vi "Stop Server.vi"(8 "error in":errorcluster, 9 "timeout ms (1000)":i32=1000, 10 "abort (F)":bool, 11 "port (0)":u16) -> (0 "error out":errorcluster)   [LabVIEW 2010, in "NI_CCC.lvlib"]
doc: "Stops the CCC server process.\n\nIf the value of <b>port</b> is 0, all instances of the CCC server process will be stopped. Otherwise, only the CCC server process instance corresponding to the port number will be stopped."
uses:
  NI_CCC.lvlib
  FG Server Instances Action.ctl
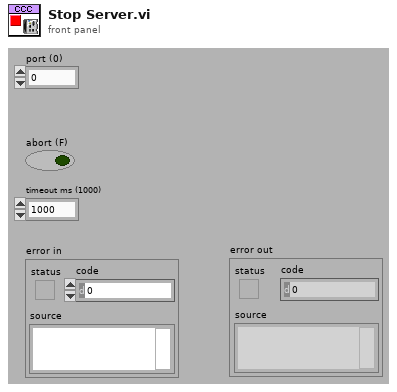
[diagram p1: front panel]
types:
  T1 = typedef "NI_CCC.lvlib/FG Server Instances Action.ctl" = enum16{"Find Instance", "Find All", "Register Instance", "Unregister Instance", "Unregister All"}
  T2 = typedef "NI_CCC.lvlib/Server Instance Data.ctl" = cluster{"server ref":refnum<vi>, "stop notifier":refnum<notifier>}
  T3 = enum32{"Bad", "Idle", "Run top level", "Running"}
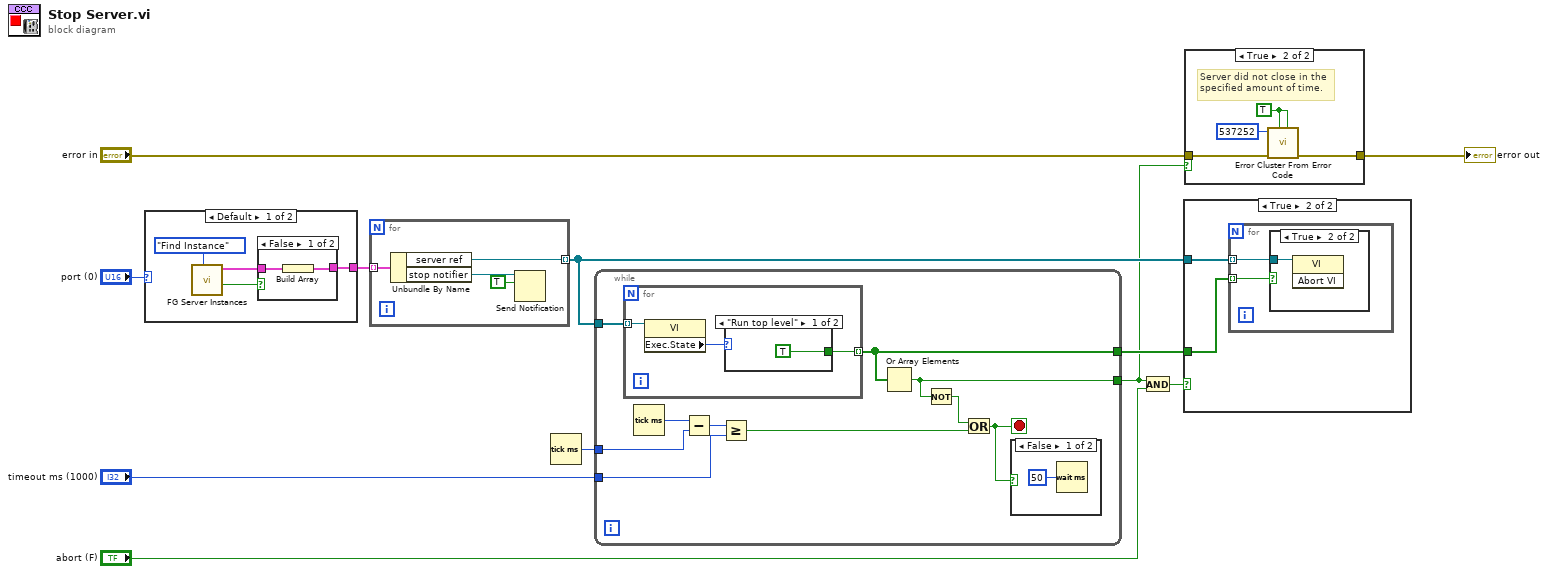
[diagram p0: block diagram]
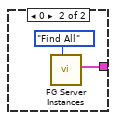
[diagram p4: hidden frame]
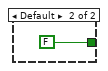
[diagram p8: hidden frame]
diagram:
  n1 = case shown="Default" "port (0)" {
    tunnel: [w12 w18] -> w5
    frame Default {
      n2 = call "FG Server Instances.vi"("action"=FG_Server_Instances_Action."Find Instance") -> ("failed?"=w14:bool, "server instance"=w13:T2)  [unwired: 7 in, 2 out]
      n3 = case shown="False" w14 {
        tunnel: w13 -> [w17 _]
        tunnel: [w16 _] -> w12
        frame False {
          n4 = Build Array(w17) -> (w16:T2[])
        }
        frame True {
        }
      }
    }
    frame 0 {
      n5 = call "FG Server Instances.vi"("action"=FG_Server_Instances_Action."Find All") -> ("all instances"=w18:T2[])  [unwired: 7 in, 3 out]
    }
  }
  n6 = for {
    tunnel: w5 -> [w23] mode=indexing
    tunnel: [w22] -> w9 mode=indexing
    n7 = Unbundle By Name(w23) -> ("server ref"=w22:refnum<vi>, "stop notifier"=w20:refnum<notifier>)
    n8 = Send Notification(notification=TRUE, notifier=w20) -> ()  [unwired: 1 in, 2 out]
  }
  n9 = Tick Count (ms)() -> (millisecond timer value=w11:u32)
  n10 = while {
    tunnel: w9 -> [w33]
    tunnel: [w32] -> w8
    tunnel: w11 -> [w29]
    tunnel: "timeout ms (1000)" -> [w28]
    tunnel: [w24] -> w1
    stop <- w25 stop-if-true
    n11 = for {
      tunnel: w33 -> [w36] mode=indexing
      tunnel: [w35] -> w32 mode=indexing
      n12 = property class="VI"(reference=w36) -> ("Exec.State"=w37:T3)  [unwired: 1 in, 2 out]
      n13 = case shown="\"Run top level\"" w37 {
        tunnel: [TRUE FALSE] -> w35
        frame "Run top level" {
        }
        frame Default {
        }
      }
    }
    n14 = Tick Count (ms)() -> (millisecond timer value=w30:u32)
    n15 = Subtract(x=w30, y=w29) -> (x-y=w31:u32)
    n16 = Greater Or Equal?(x=w31, y=w28) -> (x >= y?=w26:bool)
    n17 = Or Array Elements(Boolean array=w32) -> (logical OR=w24:bool)
    n18 = Not(x=w24) -> (.not. x?=w27:bool)
    n19 = Or(x=w27, y=w26) -> (x .or. y?=w25:bool)
    n20 = case shown="False" w25 {
      frame False {
        n21 = Wait (ms)(milliseconds to wait=u32 50) -> ()  [unwired: 1 out]
      }
      frame True {
      }
    }
  }
  n22 = And(x=w1, y="abort (F)") -> (x .and. y?=w10:bool)
  n23 = case shown="True" w10 {
    tunnel: w9 -> [_ w41]
    tunnel: w8 -> [_ w40]
    frame False {
    }
    frame True {
      n24 = for {
        tunnel: w41 -> [w43] mode=indexing
        tunnel: w40 -> [w42] mode=indexing
        n25 = case shown="True" w42 {
          tunnel: w43 -> [_ w44]
          frame False {
          }
          frame True {
            n26 = invoke class="VI" method="Abort VI"(reference=w44) -> ()  [unwired: 2 in, 3 out]
          }
        }
      }
    }
  }
  n27 = case shown="True" w1 {
    tunnel: "error in" -> [w45 w48]
    tunnel: [w45 w47] -> w2
    frame False {
    }
    frame True {
      w46 = TRUE ("show call chain? (False)")
      # "Server did not close in the specified amount of time."
      n28 = call <vilib>:"Error Cluster From Error Code.vi"("is warning? (False)"=w46, "show call chain? (False)"=w46, "error in (no error)"=w48, "error code (0)"=537252) -> ("error out"=w47:errorcluster)  [unwired: 5 out]
    }
  }
  "error out" <- w2
